vi "displayPorts.vi"   [LabVIEW 2013]
uses:
  <vilib>/NXT/Dual Mode Library/Waits/Wait_Num.vi
  <vilib>/NXT/Dual Mode Library/Advanced/NXTFlag_Get_Integer.vi
  <vilib>/NXT/Dual Mode Library/Display/drawNumber.vi
types:
  T1 = typedef "LVHSConnector.ctl" = refnum<class "BrickReference.lvclass">
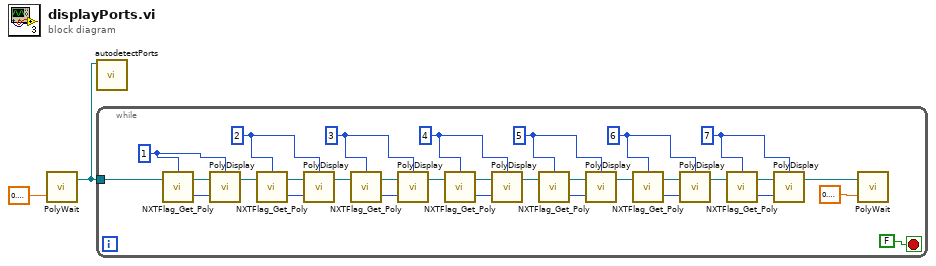
[diagram p0: block diagram]
diagram:
  n1 = call-poly <vilib>:"PolyWait.vi"("Time (1 sec)"=sgl 0.1) -> ("NXT/EV3"=w1:T1)  [unwired: 3 in]
  n2 = call "autodetectPorts.vi"("NXT/EV3"=w1) -> ()  [unwired: 11 in]
  n3 = while {
    tunnel: w1 -> [w30]
    stop <- FALSE stop-if-true
    w10 = 7 ("NXT/EV3 Flag Number")
    w11 = 6 ("NXT/EV3 Flag Number")
    w12 = 5 ("NXT/EV3 Flag Number")
    w13 = 4 ("NXT/EV3 Flag Number")
    w14 = 3 ("NXT/EV3 Flag Number")
    w15 = 2 ("NXT/EV3 Flag Number")
    w16 = 1 ("NXT/EV3 Flag Number")
    n4 = call-poly <vilib>:"NXTFlag_Get_Poly.vi"("NXT/EV3"=w30, "NXT/EV3 Flag Number"=w16) -> ("Flag Value"=w9:i32, "NXT/EV3"=w29:T1)  [unwired: 1 in]
    n5 = call-poly <vilib>:"PolyDisplay.vi"("number"=w9, "NXT/EV3"=w29, "Line"=w16) -> ("NXT/EV3"=w23:T1)  [unwired: 1 in]
    n6 = call-poly <vilib>:"NXTFlag_Get_Poly.vi"("NXT/EV3"=w23, "NXT/EV3 Flag Number"=w15) -> ("Flag Value"=w8:i32, "NXT/EV3"=w18:T1)  [unwired: 1 in]
    n7 = call-poly <vilib>:"PolyDisplay.vi"("number"=w8, "NXT/EV3"=w18, "Line"=w15) -> ("NXT/EV3"=w24:T1)  [unwired: 1 in]
    n8 = call-poly <vilib>:"NXTFlag_Get_Poly.vi"("NXT/EV3"=w24, "NXT/EV3 Flag Number"=w14) -> ("Flag Value"=w7:i32, "NXT/EV3"=w19:T1)  [unwired: 1 in]
    n9 = call-poly <vilib>:"PolyDisplay.vi"("number"=w7, "NXT/EV3"=w19, "Line"=w14) -> ("NXT/EV3"=w25:T1)  [unwired: 1 in]
    n10 = call-poly <vilib>:"NXTFlag_Get_Poly.vi"("NXT/EV3"=w25, "NXT/EV3 Flag Number"=w13) -> ("Flag Value"=w6:i32, "NXT/EV3"=w17:T1)  [unwired: 1 in]
    n11 = call-poly <vilib>:"PolyDisplay.vi"("number"=w6, "NXT/EV3"=w17, "Line"=w13) -> ("NXT/EV3"=w26:T1)  [unwired: 1 in]
    n12 = call-poly <vilib>:"NXTFlag_Get_Poly.vi"("NXT/EV3"=w26, "NXT/EV3 Flag Number"=w12) -> ("Flag Value"=w5:i32, "NXT/EV3"=w20:T1)  [unwired: 1 in]
    n13 = call-poly <vilib>:"PolyDisplay.vi"("number"=w5, "NXT/EV3"=w20, "Line"=w12) -> ("NXT/EV3"=w27:T1)  [unwired: 1 in]
    n14 = call-poly <vilib>:"NXTFlag_Get_Poly.vi"("NXT/EV3"=w27, "NXT/EV3 Flag Number"=w11) -> ("Flag Value"=w4:i32, "NXT/EV3"=w21:T1)  [unwired: 1 in]
    n15 = call-poly <vilib>:"PolyDisplay.vi"("number"=w4, "NXT/EV3"=w21, "Line"=w11) -> ("NXT/EV3"=w28:T1)  [unwired: 1 in]
    n16 = call-poly <vilib>:"NXTFlag_Get_Poly.vi"("NXT/EV3"=w28, "NXT/EV3 Flag Number"=w10) -> ("Flag Value"=w3:i32, "NXT/EV3"=w22:T1)  [unwired: 1 in]
    n17 = call-poly <vilib>:"PolyDisplay.vi"("number"=w3, "NXT/EV3"=w22, "Line"=w10) -> ("NXT/EV3"=w32:T1)  [unwired: 1 in]
    n18 = call-poly <vilib>:"PolyWait.vi"("Time (1 sec)"=sgl 0.1, "NXT/EV3"=w32) -> ()  [unwired: 2 in, 1 out]
  }
